vi "Write_Power_Off_Status.vi"(0 "Config File Ref":T1, 5 "Value":bool=TRUE, 11 "error in (no error)":errorcluster) -> (4 "Config File Ref Out":T1, 15 "error out":errorcluster)   [LabVIEW 2020]
doc: "This VI writes the last time power off status done. Wheather normal shutdown or abort done"
uses:
  <vilib>/Utility/config.llb/Config Data RefNum.ctl
  <vilib>/Utility/config.llb/Write Key (Boolean).vi
  <vilib>/Utility/config.llb/NI_LVConfig.lvlib
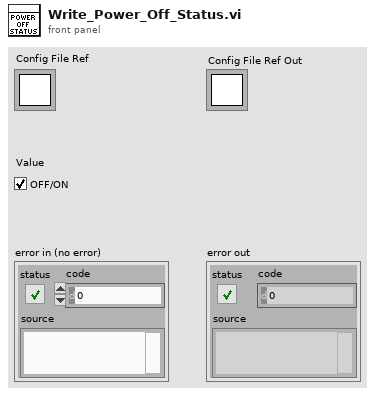
[diagram p1: front panel]
types:
  T1 = typedef "NI_LVConfig.lvlib/Config Data RefNum.ctl" = refnum<k1>
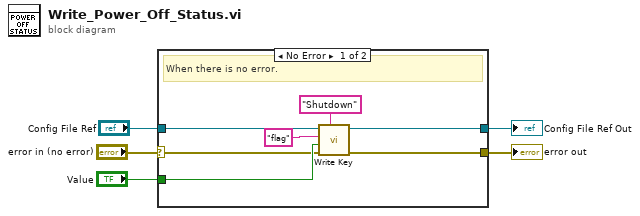
[diagram p0: block diagram]
diagram:
  n1 = case shown="No Error" "error in (no error)" {
    selector: "error in (no error)" -> [w8 w14]
    tunnel: [w9 w14] -> w5
    tunnel: "Value" -> [w12 _]
    tunnel: "Config File Ref" -> [w7 w13]
    tunnel: [w6 w13] -> w1
    frame No Error {
      # "When there is no error."
      n2 = call-poly <vilib>:"Write Key.vi"("section"="Shutdown", "error in (no error)"=w8, "value"=w12, "key"="flag", "refnum"=w7) -> ("error out"=w9:errorcluster, "refnum out"=w6:T1)  [unwired: 4 in, 1 out]
    }
    frame Error {
      # "When there is error. Do nothing"
    }
  }
  "error out" <- w5
  "Config File Ref Out" <- w1
